vi "Rescale Array.vi"(10 "Scaling Info":T1, 11 "Array to Rescale":dbl[](array[numeric])) -> (3 "Rescaled Array":dbl[](array[numeric]))   [LabVIEW 2015, in "Neural Network.lvclass"]
doc: "Apply scaling to ouptut vector."
uses:
  Neural Network.lvclass
  Types/Scaling Info.ctl
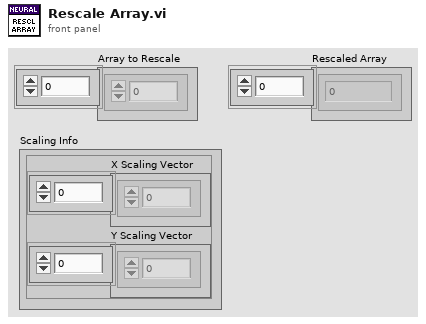
[diagram p1: front panel]
types:
  T1 = typedef "Neural Network.lvclass/Scaling Info.ctl" = cluster{"X Scaling Vector":dbl[], "Y Scaling Vector":dbl[]}
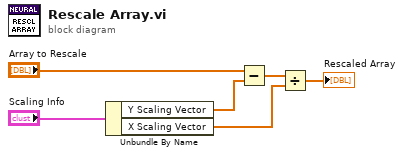
[diagram p0: block diagram]
diagram:
  n1 = Unbundle By Name("Scaling Info") -> ("Y Scaling Vector"=w1:dbl[], "X Scaling Vector"=w2:dbl[])
  n2 = Subtract(x="Array to Rescale", y=w1) -> (x-y=w4:dbl[])
  n3 = Divide(x=w4, y=w2) -> (x/y=→"Rescaled Array":dbl[])
